vi "Error Handler.vi"(8 "error in":errorcluster, 11 "queue in":refnum<queue>) -> (0 "error out":errorcluster, 3 "queue out":refnum<queue>)   [LabVIEW 2015]
doc: "This subVI monitors the Error Cluster wire running through both the Producer and Consumer Loops. The moment an Error is detected in either loop this subVI sends a message to the Consumer Loop to shut down."
uses:
  Consumer Message.ctl
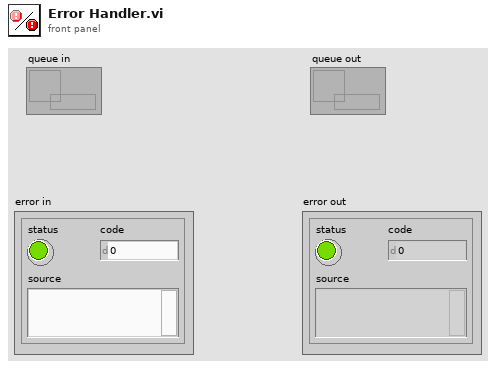
[diagram p1: front panel]
types:
  T1 = typedef "Consumer Message.ctl" = cluster{"Consumer State":string, "Boolean Data":bool, "Numeric Data":i32, "signal":dbl[], "Numeric":dbl, "Error":errorcluster}
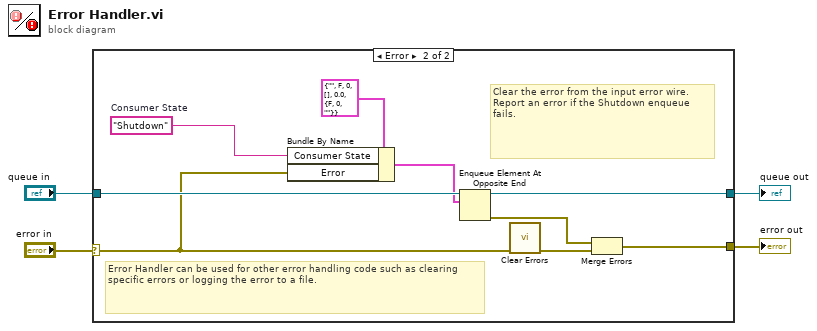
[diagram p0: block diagram]
diagram:
  n1 = case shown="Error" "error in" {
    selector: "error in" -> [w6 w10]
    tunnel: [w6 w8] -> w3
    tunnel: "queue in" -> [w5 w15]
    tunnel: [w5 w9] -> w1
    frame No Error {
    }
    frame Error {
      w11 = "Shutdown"  # Consumer State
      # "Clear the error from the input error wire. Report an error if the Shutdown enqueue fails."
      # "Error Handler can be used for other error handling code such as clearing specific errors or logging the error to a file."
      n2 = Bundle By Name(cluster=T1 {"Consumer State"="", "Boolean Data"=FALSE, "Numeric Data"=0, "signal"=[], "Numeric"=0.0, "Error"={"status"=FALSE, "code"=0, "source"=""}}, "Consumer State"=w11, "Error"=w10) -> (w14:T1)
      n3 = Enqueue Element At Opposite End(queue=w15, element=w14) -> (queue out=w9:refnum<queue>, error out=w7:errorcluster)  [unwired: 2 in, 1 out]
      n4 = call <vilib>:"Clear Errors.vi"("error in (no error)"=w10) -> ("error out"=w13:errorcluster)  [unwired: 5 in, 1 out]
      n5 = Merge Errors "Merge Errors"(w7, w13) -> (w8:errorcluster)
    }
  }
  "error out" <- w3
  "queue out" <- w1
